vi "Log Critical.vi"(8 "error in (no error)":errorcluster, 9 "error":errorcluster, 10 "Message":string, 11 "Logger in":refnum<class "Logger.lvclass">) -> (0 "error out":errorcluster, 3 "Logger out":refnum<class "Logger.lvclass">)   [LabVIEW 2017, in "Error Log.lvlib" / "Logger.lvclass"]
doc: "Logs an event with level Critical."
uses:
  Logger.lvclass
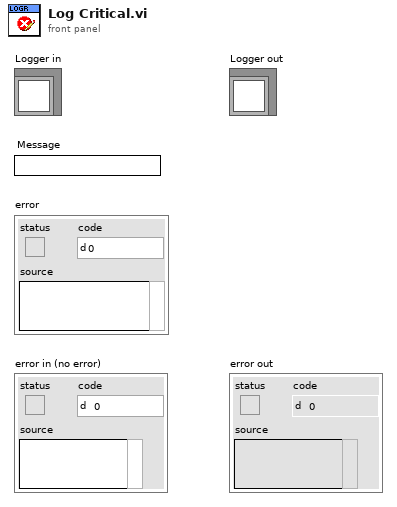
[diagram p1: front panel]
types:
  T1 = enum16{"DEBUG", "INFO", "WARNING", "ERROR", "CRITICAL"}
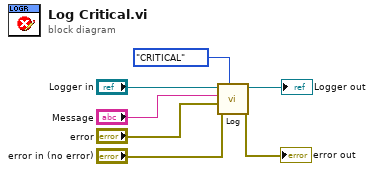
[diagram p0: block diagram]
diagram:
  n1 = call "Log.vi"("Level"=T1."CRITICAL", "error in (no error)"="error in (no error)", "error"="error", "Message"="Message", "Logger in"="Logger in") -> ("error out"=→"error out":errorcluster, "Logger out"=→"Logger out":refnum<class "Logger.lvclass">)  [unwired: 5 in]
